vi "Encoder_Noise.vi"() -> ()   [LabVIEW 2019]
panel:
  out "Measured Position(rotations)":dbl
  in  "True Position(rotations)":dbl
  in  "Position Offset Scalar":dbl
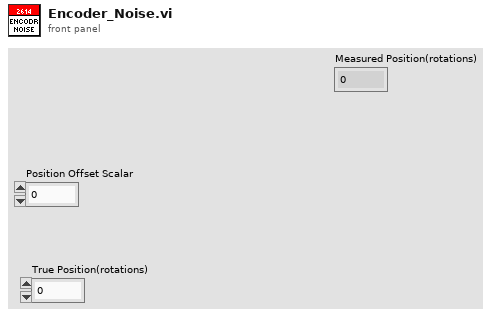
[diagram p1: front panel]
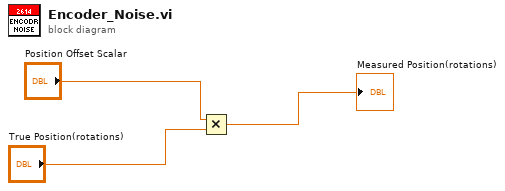
[diagram p0: block diagram]
diagram:
  n1 = Multiply(x="Position Offset Scalar", y="True Position(rotations)") -> (x*y=→"Measured Position(rotations)":dbl)
